vi "svfa_Process Coherent Output Power Subset.vi"(0 "Windowed signal [X]":waveform(dbl)={"t0"=timestamp(0 s since 1904-01-01), "dt"=1.953125e-05, "Y"=[]}, 1 "Windowed signal [Y]":waveform(dbl)={"t0"=timestamp(0 s since 1904-01-01), "dt"=1.953125e-05, "Y"=[]}, 2 "window":u16(ring) items=["None "=0, "Hanning"=1, "Hamming"=2, "Blackman-Harris"=3, "Exact Blackman"=4, "Blackman"=5, "Flat Top"=6, "4 Term B-Harris "=7, "7 Term B-Harris"=8, "Low Sidelobe"=9, "Force - Exponential"=10, "Gaussian"=62], 3 "force/exp settings":T1={"force window [%]"=50.0, "exponential window [%]"=10.0} {"exponential window [%]" min=0.0 max=100.0 format="%.2f"; "force window [%]" min=0.0 max=100.0 format="%.2f"}, 4 "averaging parameters":T10={"averaging mode"=enum."No averaging", "weighting mode"=enum."Linear", "number of averages"=10, "linear mode"=enum."Auto restart"}, 5 "error in (no error)":errorcluster, 6 "Spectrum Settings":T9 {"stop frequency" format="%.2f"; "start frequency" format="%.2f"}, 7 "processing control":T2(ring)) -> (12 "averages completed":dbl format="%.2f", 13 "processing control":T2(ring), 14 "COP":cluster{"df":dbl, "df":dbl, dbl[]} {"?" format="%.2f"; "df" format="%.2f"; "df" format="%.2f"}, 15 "coherence":cluster{"f0":dbl, "df":dbl, "coherence":dbl[]} {"coherence" format="%.2p"; "df" format="%.2p"; "f0" format="%.2p"}, 17 "averaging done":bool, 18 "spectrum info":T3={"channel name"="", "description"="", "x-axis units"=0, "spectral info"={"spectrum type"=enum."Power [Magnitude^2]", "linear/dB"=enum."linear", "window"=0, "window size"=0, "FFT size"=0}, "engineering units"=0, "custom label"="", "dB reference [EU]"=0.0, "peak units"=enum."rms", "weighting filter"=0, "spectral density?"=FALSE, "unit label"="", "spectrum skewed?"=FALSE, "complimentary spectrum units"=enum."none"} {"x-axis units" items=["Time (s)"=0, "Frequency-CB (Hz)"=1, "Frequency-CPB (Hz)"=1248, "Frequency-Arbitrary (Hz)"=2357, "Quefrency (s)"=2, "Revolutions (rev)"=3, "Order"=4, "Speed (RPM)"=11, "Speed (rad/s)"=21, "Index"=65535]; "weighting filter" items=["Linear", "A-weighting", "B-weighting", "C-weighting", "ITU-R 468-4", "Dolby", "CCITT", "C-message", "Wb", "Wc", "Wd", "We", "Wf", "Wh", "Wj", "Wk", "Wm", "AES17 20 kHz lowpass", "AES17 40 kHz lowpass", "AES17 20 kHz highpass", "AES17 40 kHz highpass"]; "dB reference [EU]" format="%.2f"; "engineering units" items=["custom..."=0, "V"=1, "A"=21, "C"=30, "pC"=31, "s"=32, "-"=29, "Pa"=2, "N"=20, "g"=3, "m/s^2"=4, "m/s"=5, "m"=6, "mm/s"=12, "mm"=13, "micron/s"=14, "micron"=15, "in/s^2"=7, "in/s"=8, "in"=9, "mil/s"=10, "mil"=11, "rad/s^2"=16, "rad/s"=17, "rad"=18, "deg/s^2"=26, "deg/s"=27, "deg"=28, "RPM"=22, "cycle/s^2"=23, "Hz"=24, "cycle"=25, "strain"=19]; "spectral info"."window" items=["None "=0, "Hanning"=1, "Hamming"=2, "Blackman-Harris"=3, "Exact Blackman"=4, "Blackman"=5, "Flat Top"=6, "4 Term B-Harris "=7, "7 Term B-Harris"=8, "Low Sidelobe"=9, "Force - Exponential"=10, "Gaussian"=62]}, 19 "error out":errorcluster)   [LabVIEW 2017]
uses:
  <vilib>/addons/_NISVFA/_Shared subVIs/Controls/svc_Spectrum Info.ctl
  <vilib>/addons/_NISVFA/_Shared subVIs/Controls/svc_X-Axis Units.ctl
  <vilib>/addons/_NISVFA/_Shared subVIs/Controls/svc_Spectrum Type.ctl
  <vilib>/addons/_NISVFA/_Shared subVIs/Controls/svc_Engineering Units Text Ring.ctl
  <vilib>/addons/_NISVFA/_Shared subVIs/Controls/svc_Weighting Filter Text Ring.ctl
  <vilib>/addons/_NISVFA/_Shared subVIs/Controls/svc_Complimentary Spectrum Units.ctl
  <vilib>/addons/_NISVFA/_Shared subVIs/Windowing/svfa_Scaled Time Domain Window (1 Ch).vi
  <vilib>/addons/_NISVFA/_Shared subVIs/Windowing/svfa_Scaled Time Domain Window (Array).vi
  <vilib>/Analysis/4window.llb/Force Window.vi
  <vilib>/Analysis/4window.llb/Force Window (DBL).vi
  <vilib>/Analysis/4window.llb/Exponential Window.vi
  <vilib>/Analysis/4window.llb/Exponential Window (DBL).vi
  <vilib>/Utility/error.llb/Error Cluster From Error Code.vi
  <vilib>/Analysis/0measdsp.llb/Scaled Time Domain Window.vi
  <vilib>/Analysis/0measdsp.llb/Scaled Time Domain Window (DBL).vi
  <vilib>/addons/_NISVFA/_Spectrum Processing/subVIs/svfa_Spectrum Info Window to windowTd Type Def.vi
  <vilib>/addons/_NISVFA/_Shared subVIs/Common/svc_Window Parameters.vi
  <vilib>/addons/_NISVFA/_Shared subVIs/Common/svc_Get Window Info.vi
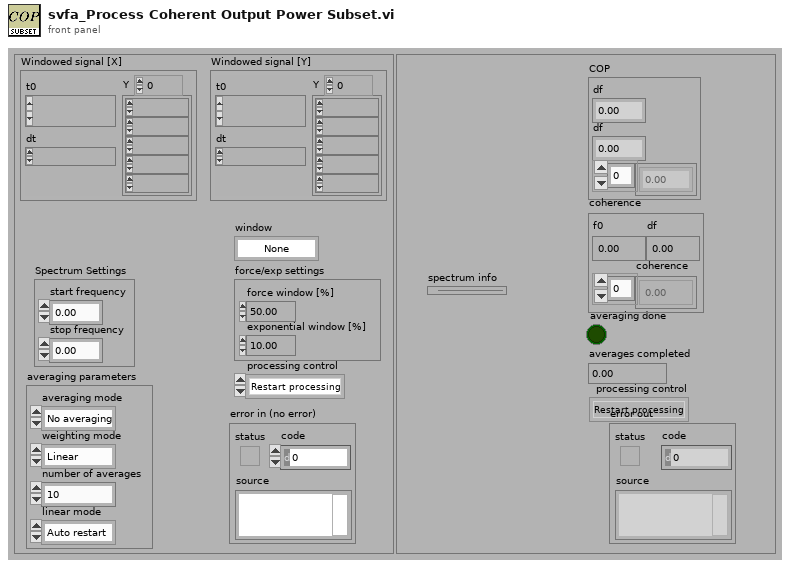
[diagram p1: front panel]
types:
  T1 = cluster{"force window [%]":dbl, "exponential window [%]":dbl}
  T2 = enum16{"Restart processing", "Continue processing", "Skip processing"}
  T3 = typedef "svc_Spectrum Info.ctl" = cluster{"channel name":string, "description":string, "x-axis units":T4, "spectral info":cluster{"spectrum type":T5, "linear/dB":enum16{"linear", "dB"}, "window":u16, "window size":i32, "FFT size":i32}, "engineering units":T6, "custom label":string, "dB reference [EU]":dbl, "peak units":enum16{"rms", "peak", "peak-peak"}, "weighting filter":T7, "spectral density?":bool, "unit label":string, "spectrum skewed?":bool, "complimentary spectrum units":T8}
  T4 = typedef "svc_X-Axis Units.ctl" = u16
  T5 = typedef "svc_Spectrum Type.ctl" = enum16{"FFT Spectrum [complex]", "Amplitude [Magnitude]", "Power [Magnitude^2]", "Cross Spectrum [complex]", "Frequency Response [Complex]"}
  T6 = typedef "svc_Engineering Units Text Ring.ctl" = u16
  T7 = typedef "svc_Weighting Filter Text Ring.ctl" = u16
  T8 = typedef "svc_Complimentary Spectrum Units.ctl" = enum16{"none", "radians", "degrees", "cycles", "imaginary"}
  T9 = cluster{"start frequency":dbl, "stop frequency":dbl}
  T10 = cluster{"averaging mode":enum16{"No averaging", "Vector averaging", "RMS averaging", "Peak hold"}, "weighting mode":enum16{"Linear", "Exponential"}, "number of averages":u32, "linear mode":enum16{"One shot", "Auto restart"}}
  T11 = typedef "svc_Window [Dual FFT].ctl" = u32
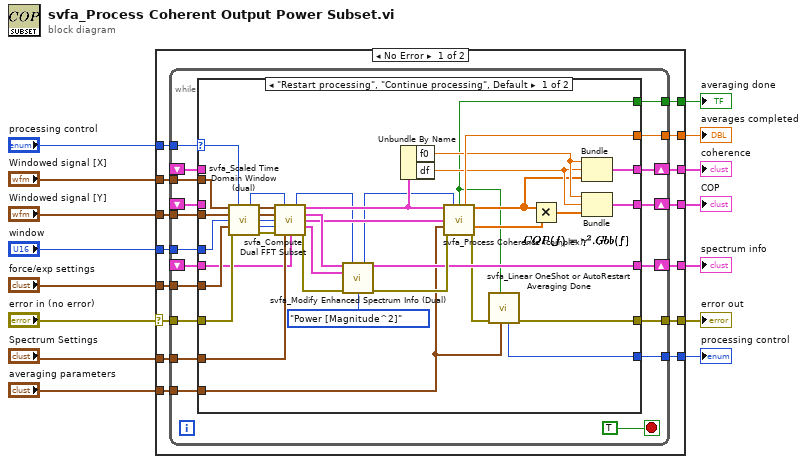
[diagram p0: block diagram]
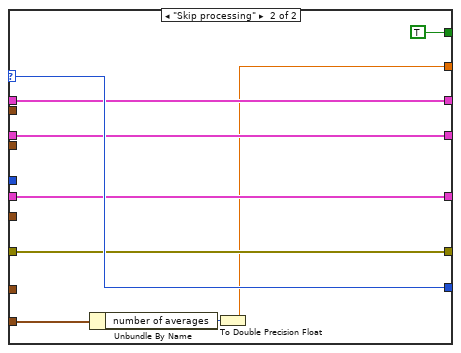
[diagram p2: hidden frame]
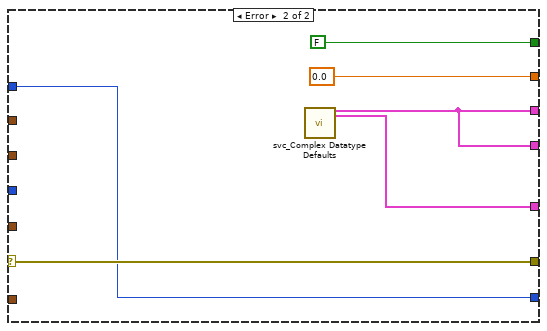
[diagram p3: hidden frame]
diagram:
  n1 = case shown="No Error" "error in (no error)" {
    selector: "error in (no error)" -> [w24 w101]
    tunnel: [w21 w101] -> w14
    tunnel: "Windowed signal [X]" -> [w28 _]
    tunnel: "Windowed signal [Y]" -> [w27 _]
    tunnel: "averaging parameters" -> [w20 _]
    tunnel: [w17 w97] -> w10
    tunnel: [w19 FALSE ("averaging done")] -> w9
    tunnel: [w30 0.0 ("averages completed")] -> w8
    tunnel: "Spectrum Settings" -> [w23 _]
    tunnel: [w18 w97] -> w6
    tunnel: "processing control" -> [w22 w98]
    tunnel: [w16 w96] -> w4
    tunnel: [w29 w98] -> w3
    tunnel: "window" -> [w26 _]
    tunnel: "force/exp settings" -> [w25 _]
    frame No Error {
      n2 = while {
        shift-left: _ -> [w32]
        shift-right: [w31] -> w16
        shift-left: _ -> [w33]
        shift-right: [w34] -> w17
        shift-left: _ -> [w35]
        shift-right: [w36] -> w18
        tunnel: [w39] -> w19
        tunnel: w20 -> [w40]
        tunnel: [w41] -> w21
        tunnel: w22 -> [w38]
        tunnel: w23 -> [w42]
        tunnel: w24 -> [w43]
        tunnel: w25 -> [w44]
        tunnel: w26 -> [w45]
        tunnel: w27 -> [w46]
        tunnel: w28 -> [w47]
        tunnel: [w48] -> w29
        tunnel: [w49] -> w30
        stop <- TRUE stop-if-true
        n3 = case shown="\"Restart processing\", \"Continue processing\", Default" w38 {
          selector: w38 -> [w55 w95]
          tunnel: [w86 w92] -> w34
          tunnel: [w85 w87] -> w49
          tunnel: [w83 w93] -> w36
          tunnel: [w78 w95] -> w48
          tunnel: w47 -> [w75 _]
          tunnel: w46 -> [w74 _]
          tunnel: w45 -> [w73 _]
          tunnel: w44 -> [w72 _]
          tunnel: w43 -> [w71 w94]
          tunnel: w42 -> [w66 _]
          tunnel: [w63 w91] -> w31
          tunnel: [w61 w94] -> w41
          tunnel: w40 -> [w59 w89]
          tunnel: [w52 TRUE ("averaging done")] -> w39
          tunnel: w35 -> [_ w93]
          tunnel: w33 -> [_ w92]
          tunnel: w32 -> [w51 w91]
          frame "Restart processing", "Continue processing", Default {
            n4 = call <vilib>:"svfa_Scaled Time Domain Window (dual).vi"("Signal in [X]"=w75, "processing control"=w55, "Signal in [Y]"=w74, "window"=w73, "force/exp settings"=w72, "error in (no error)"=w71) -> ("dup processing control"=w62:T2, "Windowed signal [X]"=w70:waveform(dbl), "Windowed signal [Y]"=w69:waveform(dbl), "window"=w65:T11, "window size"=w64:i32, "error out"=w68:errorcluster)  [unwired: 3 in, 1 out]
            n5 = call <vilib>:"svfa_Compute Dual FFT Subset.vi"("Windowed signal [X]"=w70, "processing control"=w62, "Windowed signal [Y]"=w69, "window"=w65, "window size"=w64, "error in (no error)"=w68, "Spectrum Settings"=w66, "spectrum info in"=w51) -> ("dup processing control"=w57:T2, "X FFT spectrum [Vrms]"=w79:cluster{"f0":dbl, "df":dbl, "spectrum":cdb[]}, "spectrum info X"=w82:T3, "Y FFT spectrum [Vrms]"=w58:cluster{"f0":dbl, "df":dbl, "spectrum":cdb[]}, "spectrum info Y"=w81:T3, "error out"=w84:errorcluster)  [unwired: 2 in]
            n6 = call <vilib>:"svfa_Modify Enhanced Spectrum Info (Dual).vi"("spectrum info X"=w82, "processing control"=w57, "spectrum info Y"=w81, "error in (no error)"=w84, "spectrum type"=svc_Spectrum_Type."Power [Magnitude^2]") -> ("dup processing control"=w56:T2, "spectrum info"=w63:T3, "error out"=w80:errorcluster)  [unwired: 8 in]
            n7 = Unbundle By Name(w79) -> ("f0"=w77:dbl, "df"=w76:dbl)
            n8 = call <vilib>:"svfa_Process Coherence (complex).vi"("X FFT spectrum [Vrms]"=w79, "processing control"=w56, "Y FFT spectrum [Vrms]"=w58, "averaging parameters"=w59, "error in (no error)"=w80) -> ("averaging done"=w52:bool, "averages completed"=w85:dbl, "Coherence"=w53:dbl[], "<Gyy>"=w54:dbl[], "error out"=w60:errorcluster)  [unwired: 3 in, 3 out]
            n9 = call <vilib>:"svfa_Linear OneShot or AutoRestart Averaging Done.vi"("averaging parameters"=w59, "averaging done"=w52, "error in (no error)"=w60) -> ("error out"=w61:errorcluster, "processing control"=w78:T2)  [unwired: 7 in]
            n10 = Multiply(x=w53, y=w54) -> (x*y=w67:dbl[])
            n11 = Bundle("f0"=w77, "df"=w76, "Coherence"=w53) -> (w83:cluster{"f0":dbl, "df":dbl, "Coherence":dbl[]})  [unwired: 1 in]
            n12 = Bundle("f0"=w77, "df"=w76, w67) -> (w86:cluster{"f0":dbl, "df":dbl, dbl[]})  [unwired: 1 in]
          }
          frame "Skip processing" {
            n13 = Unbundle By Name(w89) -> ("number of averages"=w88:u32)
            n14 = To Double Precision Float(number=w88) -> (double precision float=w87:dbl)
          }
        }
      }
    }
    frame Error {
      n15 = call <vilib>:"svc_Complex Datatype Defaults.vi"() -> ("empty spectrum"=w97:cluster{"f0":dbl, "df":dbl, "magnitude":dbl[]}, "dead spectrum info"=w96:T3)  [unwired: 11 in, 7 out]
    }
  }
  "error out" <- w14
  "COP" <- w10
  "averaging done" <- w9
  "averages completed" <- w8
  "spectrum info" <- w4
  "coherence" <- w6
  "processing control" <- w3
